vi "Project Parser_Map Array.vi"(7 "To Lower Case?(T)":bool=TRUE, 8 "Error In":errorcluster, 9 "External Targets":T3[](array[typedef]), 10 "Internal Targets":T2[](array[typedef]), 11 "Project Path in":path) -> (0 "Error Out":errorcluster, 1 "Found External Dependencies":T1[](array[typedef]), 2 "Found Internal Dependencies":T1[](array[typedef]), 3 "Project Path dub":path)   [LabVIEW 2019, in "Project.Dependencies Finder.lvlib"]
doc: "Parse a project file for internal and external dependencies.\n\nInternal dependencies are expected to have 'paths' like vi.lib\\ and should be found inside the LabVIEW folder.\nExternal dependencies are identified by unique folder names.\n\n2020-11-11: Henrik Dueholm Hansen"
uses:
  Project.Dependencies Finder.lvlib
  Ctl/Ctl_External Target Element.ctl
  Ctl/Ctl_Internal Target Element.ctl
  Ctl/Ctl_Dependency Element.ctl
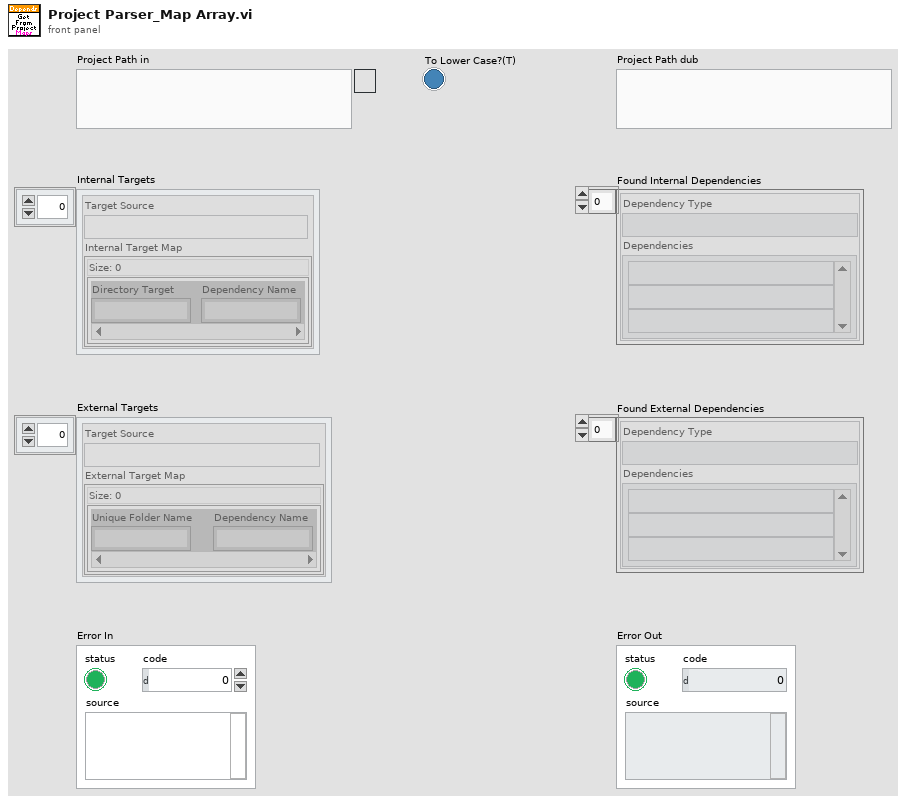
[diagram p1: front panel]
types:
  T1 = typedef "Project.Dependencies Finder.lvlib/Ctl_Dependency Element.ctl" = cluster{"Dependency Type":string, "Dependencies":string[]}
  T2 = typedef "Project.Dependencies Finder.lvlib/Ctl_Internal Target Element.ctl" = cluster{"Target Source":string, "Internal Target Map":map{string, string}}
  T3 = typedef "Project.Dependencies Finder.lvlib/Ctl_External Target Element.ctl" = cluster{"Target Source":string, "External Target Map":map{string, string}}
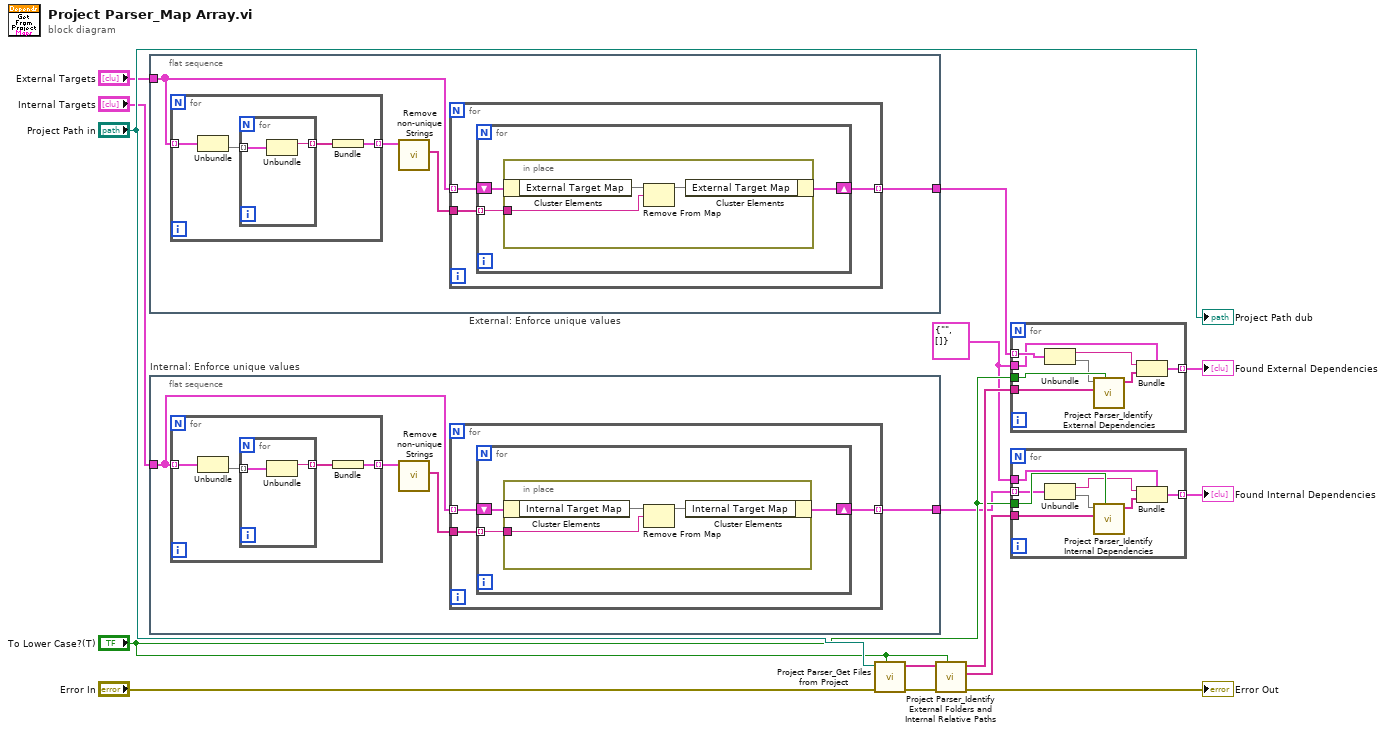
[diagram p0: block diagram]
diagram:
  w8 = T1 {"Dependency Type"="", "Dependencies"=[]} ("External Target Element")
  n1 = flat-sequence "External: Enforce unique values" {
    tunnel: "External Targets" -> [w17]
    tunnel: [w16] -> w4
    frame #0 {
      n2 = for {
        tunnel: w17 -> [w32] mode=indexing
        tunnel: [w29] -> w19 mode=indexing
        n3 = Unbundle(w32) -> ("External Target Map"=w31:map{string, string})  [unwired: 1 out]
        n4 = for {
          tunnel: w31 -> [w34] mode=indexing
          tunnel: [w33] -> w30 mode=indexing
          n5 = Unbundle(w34) -> ("Unique Folder Name"=w33:string)  [unwired: 1 out]
        }
        n6 = Bundle(w30) -> (w29:cluster{string[]})  [unwired: 1 in]
      }
      n7 = call "Remove non-unique Strings.vi"("String Array in"=w19) -> ("Removed Strings"=w18:string[])  [unwired: 9 in, 1 out]
      n8 = for {
        tunnel: w18 -> [w21]
        tunnel: w17 -> [w22] mode=indexing
        tunnel: [w20] -> w16 mode=indexing
        n9 = for {
          tunnel: w21 -> [w23] mode=indexing
          shift-right: [w24] -> w20
          shift-left: w22 -> [w25]
          n10 = in-place {
            in-place-border: w23 -> [w27]
            n11 = in-place-cluster #1(w25) -> ("External Target Map"=w28:map{string, string})
            n12 = Remove From Map(10:w27, 11:w28) -> (3:w26:map{string, string})  [unwired: 2 out]
            n13 = in-place-cluster #1("External Target Map"=w26) -> (w24:T3)
          }
        }
      }
    }
  }
  n14 = flat-sequence "Internal: Enforce unique values" {
    tunnel: "Internal Targets" -> [w36]
    tunnel: [w35] -> w2
    frame #0 {
      n15 = for {
        tunnel: w36 -> [w51] mode=indexing
        tunnel: [w48] -> w37 mode=indexing
        n16 = Unbundle(w51) -> ("Internal Target Map"=w50:map{string, string})  [unwired: 1 out]
        n17 = for {
          tunnel: w50 -> [w53] mode=indexing
          tunnel: [w52] -> w49 mode=indexing
          n18 = Unbundle(w53) -> ("Directory Target"=w52:string)  [unwired: 1 out]
        }
        n19 = Bundle(w49) -> (w48:cluster{string[]})  [unwired: 1 in]
      }
      n20 = call "Remove non-unique Strings.vi"("String Array in"=w37) -> ("Removed Strings"=w38:string[])  [unwired: 9 in, 1 out]
      n21 = for {
        tunnel: w38 -> [w39]
        tunnel: w36 -> [w41] mode=indexing
        tunnel: [w40] -> w35 mode=indexing
        n22 = for {
          tunnel: w39 -> [w42] mode=indexing
          shift-right: [w43] -> w40
          shift-left: w41 -> [w44]
          n23 = in-place {
            in-place-border: w42 -> [w46]
            n24 = in-place-cluster #2(w44) -> ("Internal Target Map"=w47:map{string, string})
            n25 = Remove From Map(10:w46, 11:w47) -> (3:w45:map{string, string})  [unwired: 2 out]
            n26 = in-place-cluster #2("Internal Target Map"=w45) -> (w43:T2)
          }
        }
      }
    }
  }
  n27 = call "Project Parser_Get Files from Project.vi"("To Lower Case?(T)"="To Lower Case?(T)", "error in (no error)"="Error In", "Project Path"="Project Path in") -> ("error out"=w13:errorcluster, "Project Files"=w1:string[])  [unwired: 6 in, 1 out]
  n28 = call "Project Parser_Identify External Folders and Internal Relative Paths.vi"("To Lower Case?(T)"="To Lower Case?(T)", "error in (no error)"=w13, "Project Files"=w1) -> ("error out"=→"Error Out":errorcluster, "Internal Relative Paths"=w10:string[], "External Folder Combinations"=w11:string[])  [unwired: 6 in]
  n29 = for {
    tunnel: w11 -> [w61]
    tunnel: "To Lower Case?(T)" -> [w60]
    tunnel: w4 -> [w59] mode=indexing
    tunnel: w8 -> [w57]
    tunnel: [w54] -> w7 mode=indexing
    n30 = Unbundle(w59) -> ("Target Source"=w56:string, "External Target Map"=w58:map{string, string})
    n31 = call "Project Parser_Identify External Dependencies.vi"("To Lower Case?(T)"=w60, "External Folder Names"=w61, "External Target Map"=w58) -> ("Found External Dependencies"=w55:string[])  [unwired: 8 in]
    n32 = Bundle(cluster=w57, "Dependency Type"=w56, "Dependencies"=w55) -> (w54:T1)
  }
  "Found External Dependencies" <- w7
  n33 = for {
    tunnel: w10 -> [w69]
    tunnel: "To Lower Case?(T)" -> [w68]
    tunnel: w2 -> [w67] mode=indexing
    tunnel: w8 -> [w65]
    tunnel: [w62] -> w6 mode=indexing
    n34 = Unbundle(w67) -> ("Target Source"=w64:string, "Internal Target Map"=w66:map{string, string})
    n35 = call "Project Parser_Identify Internal Dependencies.vi"("To Lower Case?(T)"=w68, "Internal Relative Paths"=w69, "Internal Target Map"=w66) -> ("Found Internal Dependencies"=w63:string[])  [unwired: 8 in]
    n36 = Bundle(cluster=w65, "Dependency Type"=w64, "Dependencies"=w63) -> (w62:T1)
  }
  "Found Internal Dependencies" <- w6
  "Project Path dub" <- "Project Path in"
